vi "broadcastReg-UnitTest.vi"() -> (3 "Pass?":bool)   [LabVIEW 2017, in "testcase-Broadcast Registry.lvclass"]
uses:
  testcase-Broadcast Registry.lvclass
panel:
  in  "Array":T1(array[cluster])=[{"status"="status@source >> api@target -><register>\n", "Response Message Info"=["api"], TRUE, "Response Message Info 2"=["api"]}, {"status"="status@* >> api@target -><register>", "Response Message Info"=["api"], TRUE, "Response Message Info 2"=["api"]}, {"status"="status@source >> api@target -><register>\nstatus@source >> api2@target -><register>\nstatus@source >> api@target -><unregister>", "Response Message Info"=["api2"], TRUE, "Response Message Info 2"=["api2"]}, {"status"="status@source >> api@target -><register>\nstatus@source >> api2@target -><register>\nstatus@source >> api3@target -><register>\n", "Response Message Info"=["api", "api2", "api3"], TRUE, "Response Message Info 2"=["api", "api2", "api3"]}, {"status"="status@* >> api@target -><register>\nstatus@source >> api2@target -><register>", "Response Message Info"=["api2", "api"], TRUE, "Response Message Info 2"=["api2", "api"]}, {"status"="status@* >> api@target -><register>\nstatus@source >> api@target -><unregister>", "Response Message Info"=[], TRUE, "Response Message Info 2"=[]}, {"status"="status@source >> api@target -><register>\nstatus@source >> api2@target -><register>\nstatus@source >> api@target2 -><register>", "Response Message Info"=["api", "api2"], TRUE, "Response Message Info 2"=["api", "api2"]}, {"status"="status@* >> api@target -><register>\nstatus@source >> api@target -><register>", "Response Message Info"=["api"], TRUE, "Response Message Info 2"=["api"]}, {"status"="status@* >> api@target -><register>\nstatus@source >> api@target -><register>\nstatus@* >> api@target -><unregister>", "Response Message Info"=[], TRUE, "Response Message Info 2"=[]}, {"status"="status@source >> api@target2 -><register>\nstatus@source >> api2@target2 -><register>\nstatus@source >> api@target -><register>", "Response Message Info"=["api"], TRUE, "Response Message Info 2"=["api"]}, {"status"="status@source >> api@target2 -><register>\nstatus@source >> api2@target2 -><register>\nstatus@source >> api1@target -><register>\nstatus@source >> api2@target -><register>", "Response Message Info"=["api1", "api2"], TRUE, "Response Message Info 2"=["api1", "api2"]}, {"status"="status@source >> api@target2 -><register>\nstatus@source >> api2@target2 -><register>\nstatus@source >> api1@target -><register>\nstatus@source >> api2@target -><register>\nstatus@source >> api1@target -><unregister>", "Response Message Info"=["api2"], TRUE, "Response Message Info 2"=["api2"]}, {"status"="status@source >> api@target2 -><register>\nstatus@source >> api2@target2 -><register>\nstatus@source >> api1@target -><register>\nstatus@source >> api2@target -><register>\nstatus@source >> api2@target -><unregister>", "Response Message Info"=["api1"], TRUE, "Response Message Info 2"=["api1"]}, {"status"="status@source >> api@target2 -><register>\nstatus@source >> api2@target2 -><register>\nstatus@source >> api1@target -><register>\nstatus@source >> api2@target -><register>\nstatus@* >> api2@target -><unregister>", "Response Message Info"=["api1"], TRUE, "Response Message Info 2"=["api1"]}, {"status"="status@source >> api1@target -><register>\nstatus@source >> api2@target -><register>\nstatus@* >> api2@target -><unregister>", "Response Message Info"=["api1"], TRUE, "Response Message Info 2"=["api1"]}, {"status"="status@source >> api@target2 -><register>\nstatus@source2 >> api2@target2 -><register>\nstatus@source >> api1@target -><register>\nstatus@source2 >> api1@target -><register>\nstatus@* >> api1@target -><unregister>", "Response Message Info"=[], TRUE, "Response Message Info 2"=[]}, {"status"="status@source >> api@target2 -><register>\nstatus@source2 >> api2@target2 -><register>\nstatus@source >> api1@target -><register>\nstatus@source2 >> api1@target -><register>\nstatus@source2 >> api1@target -><unregister>", "Response Message Info"=["api1"], TRUE, "Response Message Info 2"=["api1"]}, {"status"="status@source >> api@target -><register>\nstatus@source2 >> api2@target -><register>\nstatus@source -><unregister>", "Response Message Info"=["api"], TRUE, "Response Message Info 2"=["api"]}, {"status"="status@source >> api@target -><register>\nstatus@source2 >> api2@target -><register>\nstatus@* >>  api@target -><unregister>", "Response Message Info"=[], TRUE, "Response Message Info 2"=[]}, {"status"="status@source >> api@target -><register>\nstatus@source2 >> api2@target -><register>\nstatus@* >>  api@target -><unregister>", "Response Message Info"=[], FALSE, "Response Message Info 2"=["api"]}, {"status"="status@source >> api@target -><register>\nstatus@source2 >> api2@target -><register>\nstatus@* >>  api2@target -><unregister>", "Response Message Info"=["api"], TRUE, "Response Message Info 2"=["api"]}, {"status"="status@source >> api@target -><register>\nstatus@source2 >> api2@target -><register>\nstatus@* >>  *@target -><unregister>", "Response Message Info"=[], TRUE, "Response Message Info 2"=[]}, {"status"="status@source >> api@target -><register>\nstatus@source2 >> api2@target -><register>\nstatus@* >>  *@target -><unregister>", "Response Message Info"=[], TRUE, "Response Message Info 2"=[]}, {"status"="status@* >> api@target -><register>\nstatus@source >> api@target -><unregister>", "Response Message Info"=[], TRUE, "Response Message Info 2"=[]}, {"status"="status@* >> api@target -><register>\nstatus@source >> api@target -><unregister>\nstatus@* >> target -><unregister>", "Response Message Info"=[], TRUE, "Response Message Info 2"=[]}, {"status"="status@source >> api@target -><register>\nstatus@source2 >> api2@target -><register>\nstatus@* >>  api2@target -><unregister>", "Response Message Info"=["api"], TRUE, "Response Message Info 2"=["api"]}]
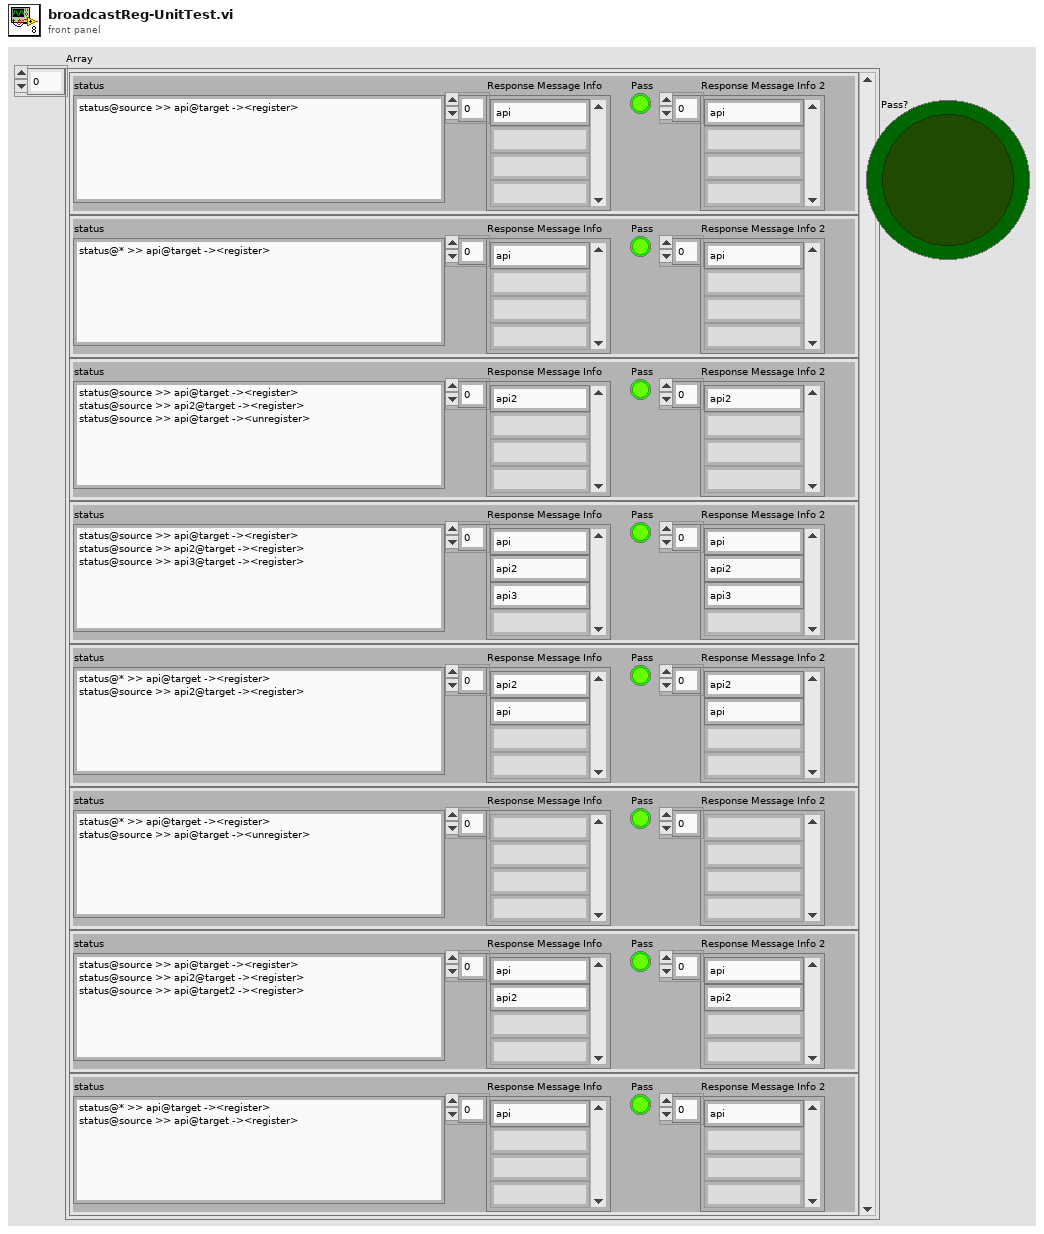
[diagram p1: front panel]
types:
  T1 = cluster{"status":string, "Response Message Info":string[], bool, "Response Message Info 2":string[]}[]
  T2 = typedef "Communicable State Machine.lvlib/BroadcastRegistry-Value.ctl" = cluster{"Name":string, "Priority":T3}
  T3 = typedef "Communicable State Machine.lvlib/CSM - Broadcast Message Type.ctl" = enum16{"Status", "Interrupt"}
  T4 = cluster{"status":string, "Response Message Info":string[], bool, "Response Message Info 2":string[]}
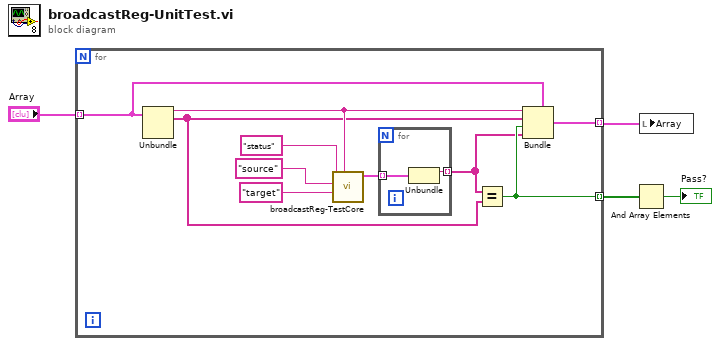
[diagram p0: block diagram]
diagram:
  n1 = for {
    tunnel: "Array" -> [w9] mode=indexing
    tunnel: [w10] -> w3 mode=indexing
    tunnel: [w7] -> w2 mode=indexing
    n2 = Unbundle(w9) -> ("status"=w11:string, "Response Message Info"=w8:string[])  [unwired: 2 out]
    n3 = call "broadcastReg-TestCore.vi"("status"=w11, "Target"="target", "Source"="source", "Status"="status") -> ("Response Message Info"=w6:T2[])  [unwired: 7 in]
    n4 = for {
      tunnel: w6 -> [w16] mode=indexing
      tunnel: [w15] -> w5 mode=indexing
      n5 = Unbundle(w16) -> ("Name"=w15:string)  [unwired: 1 out]
    }
    n6 = Equal?(x=w5, y=w8) -> (x = y?=w7:bool)
    n7 = Bundle(cluster=w9, "status"=w11, "Response Message Info"=w8, w7, "Response Message Info 2"=w5) -> (w10:T4)
  }
  n8 = And Array Elements(Boolean array=w2) -> (logical AND=→"Pass?":bool)
  n9 = local write "Array"(w3) -> ()
